vi "Create Message Data Clusters (simple).vi"(8 "error in (no error)":errorcluster, 10 "Message Metadata":T1, 11 "Library":refnum<vi>) -> (0 "error out":errorcluster, 3 "Library":refnum<vi>)   [LabVIEW 2019, in "gRPC Template Creation Utility.lvlib"]
uses:
  gRPC Template Creation Utility.lvlib
  TypeDefs/Message Metadata (Scripting).ctl
  TypeDefs/Message Element Metadata (Scripting).ctl
  TypeDefs/Message Element Type.ctl
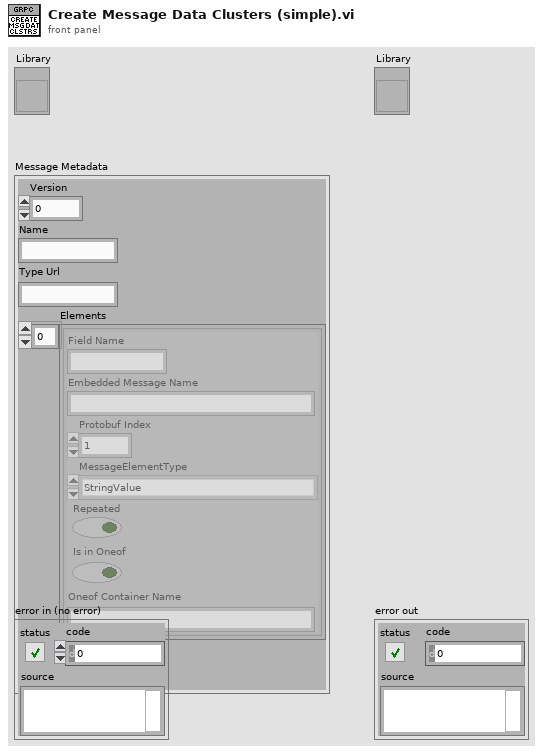
[diagram p1: front panel]
types:
  T1 = typedef "gRPC Template Creation Utility.lvlib/Message Metadata (Scripting).ctl" = cluster{"Version":i32, "Name":string, "Type Url":string, "Elements":T2[], "Has Oneof":bool}
  T2 = typedef "gRPC Template Creation Utility.lvlib/Message Element Metadata (Scripting).ctl" = cluster{"Field Name":string, "Embedded Message Name":string, "Protobuf Index":i32, "MessageElementType":T3, "Repeated":bool, "Is in Oneof":bool, "Oneof Container Name":string}
  T3 = typedef "gRPC Template Creation Utility.lvlib/Message Element Type.ctl" = enum32{"Int32Value", "FloatValue", "DoubleValue", "BoolValue", "StringValue", "MessageValue", "Int64Value", "UInt32Value", "UInt64Value", "EnumValue", "Bytes", "Fixed64", "Fixed32", "SFixed64", "SFixed32", "SInt64", "SInt32", "Oneof"}
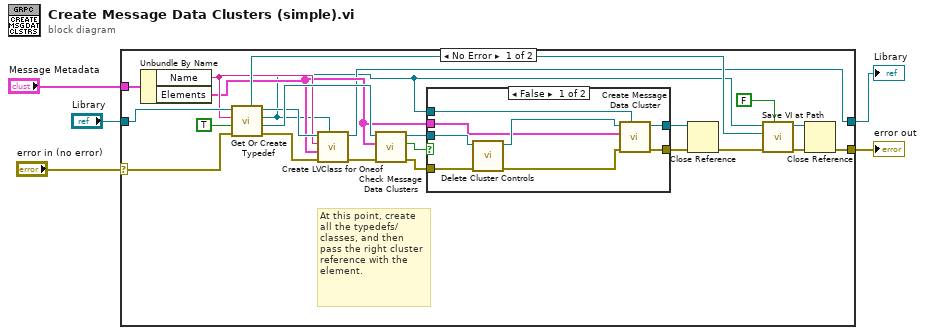
[diagram p0: block diagram]
diagram:
  n1 = case shown="No Error" "error in (no error)" {
    selector: "error in (no error)" -> [w24 w39]
    tunnel: "Message Metadata" -> [w28 _]
    tunnel: "Library" -> [w27 w40]
    tunnel: [w16 w39] -> w3
    tunnel: [w8 w40] -> w2
    frame No Error {
      # "At this point, create all the typedefs/classes, and then\npass the right cluster reference with the element."
      n2 = Unbundle By Name(w28) -> ("Name"=w11:string, "Elements"=w10:T2[])
      n3 = call "Get Or Create Typedef.vi"("error in (no error)"=w24, "Create cluster inside Typedef?"=TRUE, "Name"=w11, "Library in"=w27) -> ("error out"=w9:errorcluster, "Cluster ref out"=w15:refnum<vi>, "VI ref out"=w6:refnum<vi>, "Library out"=w12:refnum<vi>, "Path"=w14:path)  [unwired: 3 in]
      n4 = call "Create LVClass for Oneof.vi"("Parent Message Typedef"=w6, "error in (no error)"=w9, "Message Elements"=w10, "Message Name"=w11, "Library"=w12) -> ("error out"=w7:errorcluster, "Library"=w8:refnum<vi>)  [unwired: 5 in]
      n5 = call "Check Message Data Clusters.vi"("error in (no error)"=w7, "Fields Data"=w10, "Message Data Cluster in"=w15) -> ("error out"=w17:errorcluster, "Unmodified?"=w18:bool, "Message Data Cluster out"=w19:refnum<vi>)  [unwired: 6 in]
      n6 = case shown="False" w18 {
        tunnel: [w36 w37] -> w23
        tunnel: w17 -> [w34 w37]
        tunnel: w19 -> [w33 w38]
        tunnel: [w31 w38] -> w21
        tunnel: w10 -> [w30 _]
        tunnel: w6 -> [w29 _]
        frame False {
          n7 = call "Delete Cluster Controls.vi"("error in (no error)"=w34, "Cluster in"=w33) -> ("error out"=w35:errorcluster, "Cluster out"=w32:refnum<vi>)  [unwired: 8 in]
          n8 = call "Create Message Data Cluster.vi"("Owning vi ref (typeDef)"=w29, "error in (no error)"=w35, "Message Elements MetaData"=w30, "Cluster ref in"=w32) -> ("error out"=w36:errorcluster, "Cluster ref out"=w31:refnum<vi>)  [unwired: 6 in]
        }
        frame True {
        }
      }
      n9 = Close Reference(reference=w21, error in (no error)=w23) -> (error out=w22:errorcluster)
      n10 = call "Save VI at Path.vi"("Override Existing? (T)"=FALSE, "error in (no error)"=w22, "Path"=w14, "VI in"=w6) -> ("error out"=w26:errorcluster, "VI out"=w25:refnum<vi>)  [unwired: 5 in, 1 out]
      n11 = Close Reference(reference=w25, error in (no error)=w26) -> (error out=w16:errorcluster)
    }
    frame Error {
    }
  }
  "error out" <- w3
  "Library" <- w2
